vi "DAQ- Steper 2.vi"(0 "Travel (Degree)":dbl=100.0, 5 "Mode":i32(ring)=10178 items=["Finite Samples"=10178, "Continuous Samples"=10123, "Hardware Timed Single Point"=12522], 7 "Home Done":bool, 9 "Speed d/s":dbl=10.0, 11 "error in":errorcluster) -> (6 "Task Done Bit":bool, 15 "error out":errorcluster)   [LabVIEW 2015]
uses:
  Project Setup/Globle Variable/GR_Servo.vi
  <vilib>/DAQmx/create/channels.llb/DAQmx Create Channel (CO-Pulse Generation-Frequency).vi
  <vilib>/DAQmx/configure/timing.llb/DAQmx Timing (Implicit).vi
  Galobal variable_TI.vi
panel:
  out "32bit integer":i32
  in  "Motor PPR":dbl=3600.0
  in  "Motor Gear Ratio":dbl=1.0
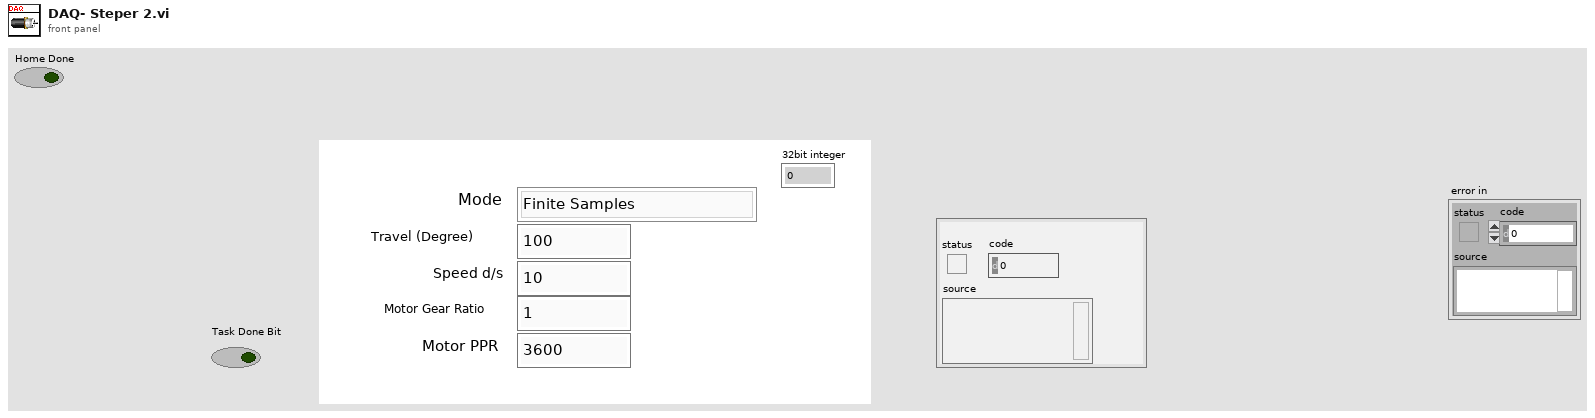
[diagram p1: front panel]
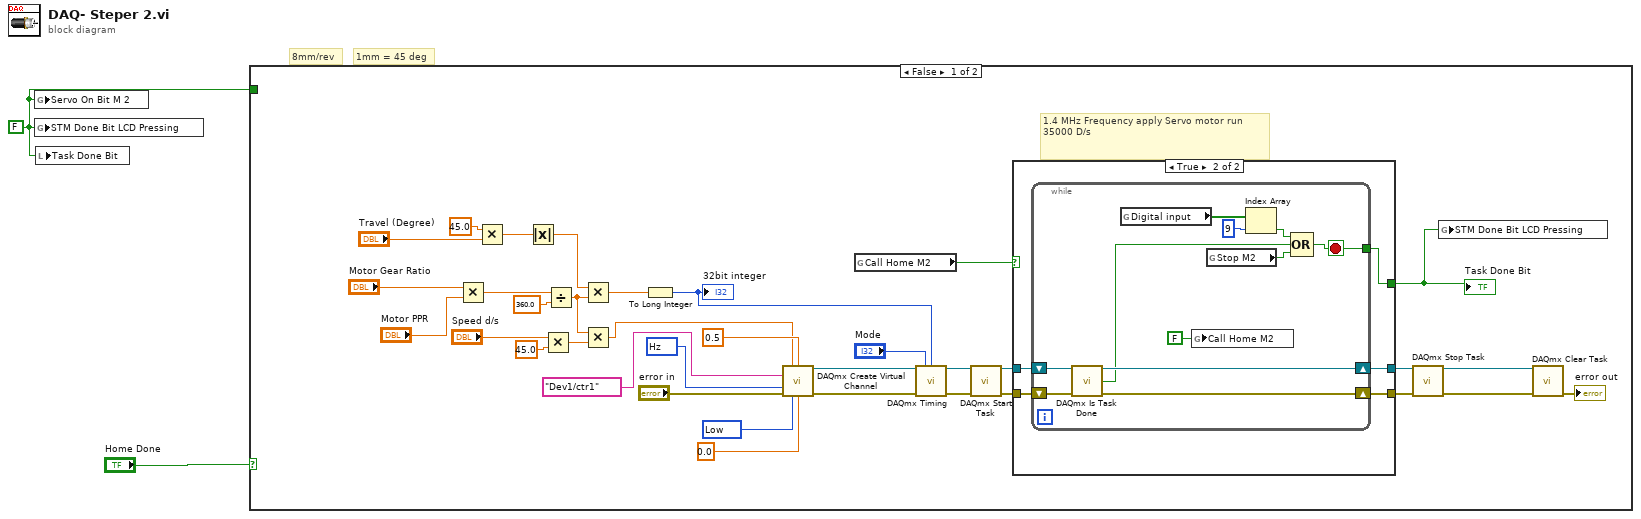
[diagram p0: block diagram]
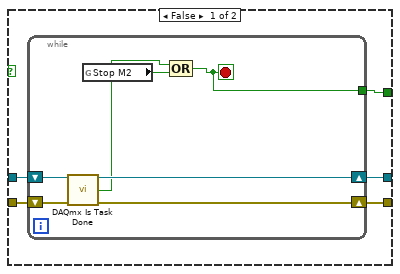
[diagram p2: hidden frame]
diagram:
  w2 = FALSE ("Servo On Bit M 2")
  # "1mm = 45 deg"
  # "8mm/rev"
  n1 = global write "GR_Servo.vi" "Servo On Bit M 2"(w2) -> ()
  n2 = global write "GR_Servo.vi" "STM Done Bit LCD Pressing"(w2) -> ()
  n3 = local write "Task Done Bit"(w2) -> ()
  n4 = case shown="False" "Home Done" {
    tunnel: w2 -> [_ _]
    frame False {
      w16 = 10373 items=["Hz"=10373] ("units")
      w17 = 10214 items=["High"=10192, "Low"=10214] ("idle state")
      # "1.4 MHz Frequency apply Servo motor run \n35000 D/s"
      n5 = Multiply(x="Motor Gear Ratio", y="Motor PPR") -> (x*y=w26:dbl)
      n6 = Multiply(x=45.0, y="Travel (Degree)") -> (x*y=w14:dbl)
      n7 = Absolute Value(x=w14) -> (abs(x)=w25:dbl)
      n8 = Multiply(x="Speed d/s", y=45.0) -> (x*y=w11:dbl)
      n9 = Divide(x=w26, y=360.0) -> (x/y=w30:dbl)
      n10 = Multiply(x=w25, y=w30) -> (x*y=w15:dbl)
      n11 = Multiply(x=w30, y=w11) -> (x*y=w34:dbl)
      n12 = To Long Integer(number=w15) -> (32bit integer=w37:i32)
      "32bit integer" <- w37
      n13 = call-poly <vilib>:"DAQmx Create Virtual Channel.vi"("frequency"=w34, "duty cycle"=0.5, "counter"=tag "Dev1/ctr1", "units"=w16, "error in"="error in", "idle state"=w17, "initial delay"=0.0) -> ("task out"=w19:refnum<k21>, "error out"=w20:errorcluster)  [unwired: 7 in]
      n14 = global read "Galobal variable_TI.vi" "Call Home M2"() -> (w6:bool)
      n15 = call-poly <vilib>:"DAQmx Timing.vi"("task/channels in"=w19, "sample mode"="Mode", "samples per channel"=w37, "error in"=w20) -> ("task out"=w21:refnum<k21>, "error out"=w22:errorcluster)  [unwired: 10 in]
      n16 = call <vilib>:"DAQmx Start Task.vi"("task/channels in"=w21, "error in"=w22) -> ("task out"=w8:refnum<k21>, "error out"=w7:errorcluster)  [unwired: 12 in]
      n17 = case shown="True" w6 {
        tunnel: [w42 w51] -> w4
        tunnel: w8 -> [w41 w54]
        tunnel: [w40 w52] -> w5
        tunnel: w7 -> [w39 w53]
        tunnel: [w38 w50] -> w3
        frame False {
          n18 = while {
            shift-right: [w47] -> w40
            shift-left: w41 -> [w49]
            shift-right: [w48] -> w42
            shift-left: w39 -> [w46]
            tunnel: [w43] -> w38
            stop <- w43 stop-if-true
            n19 = call <vilib>:"DAQmx Is Task Done.vi"("task/channels in"=w49, "error in"=w46) -> ("task out"=w47:refnum<k21>, "task done?"=w44:bool, "error out"=w48:errorcluster)  [unwired: 11 in]
            n20 = global read "Galobal variable_TI.vi" "Stop M2"() -> (w45:bool)
            n21 = Compound Arithmetic op=OR(w44, w45) -> (w43:bool)
          }
        }
        frame True {
          n22 = while {
            shift-right: [w63] -> w52
            shift-left: w54 -> [w65]
            shift-right: [w64] -> w51
            shift-left: w53 -> [w62]
            tunnel: [w56] -> w50
            stop <- w56 stop-if-true
            n23 = call <vilib>:"DAQmx Is Task Done.vi"("task/channels in"=w65, "error in"=w62) -> ("task out"=w63:refnum<k21>, "task done?"=w58:bool, "error out"=w64:errorcluster)  [unwired: 11 in]
            n24 = global read "Galobal variable_TI.vi" "Digital input"() -> (w59:bool[])
            n25 = global write "Galobal variable_TI.vi" "Call Home M2"(FALSE ("Call Home M2")) -> ()
            n26 = global read "Galobal variable_TI.vi" "Stop M2"() -> (w61:bool)
            n27 = Index Array(array=w59, index=9) -> (element=w57:bool)
            n28 = Compound Arithmetic op=OR(w57, w58, w61) -> (w56:bool)
          }
        }
      }
      "Task Done Bit" <- w3
      n29 = call <vilib>:"DAQmx Stop Task.vi"("task/channels in"=w5, "error in"=w4) -> ("task out"=w23:refnum<k21>, "error out"=w33:errorcluster)  [unwired: 12 in]
      n30 = global write "GR_Servo.vi" "STM Done Bit LCD Pressing"(w3) -> ()
      n31 = call <vilib>:"DAQmx Clear Task.vi"("task in"=w23, "error in"=w33) -> ("error out"=→"error out":errorcluster)  [unwired: 13 in]
    }
    frame True {
    }
  }
